vi "Administrator.vi"(10 "string":string="001001/12345:67890") -> (2 "on/off":bool)   [LabVIEW 2011]
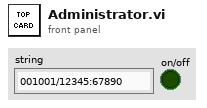
[diagram p1: front panel]
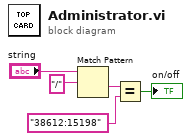
[diagram p0: block diagram]
diagram:
  n1 = Match Pattern(string="string", regular expression="/") -> (after substring=w3:string)  [unwired: 1 in, 3 out]
  n2 = Equal?(x=w3, y="38612:15198") -> (x = y?=→"on/off":bool)
